vi "Read Response Simple.vi"(7 "output file":path, 8 "error in (no error)":errorcluster, 11 "HttpResponseMessage in":refnum<class "HttpResponseMessage.lvclass">) -> (0 "error out":errorcluster, 1 "Response":string, 2 "Headers":T1, 4 "Timeout":bool, 5 "StatusCode":i32(ring)=100 items=["Continue"=100, "SwitchingProtocols"=101, "OK"=200, "Created"=201, "Accepted"=202, "NonAuthoritativeInformation"=203, "NoContent"=204, "ResetContent"=205, "PartialContent"=206, "MultipleChoices, Ambiguous"=300, "MovedPermanently, Moved"=301, "Found, Redirect"=302, "SeeOther, RedirectMethod"=303, "NotModified"=304, "UseProxy"=305, "Unused"=306, "TemporaryRedirect, RedirectKeepVerb"=307, "BadRequest"=400, "Unauthorized"=401, "PaymentRequired"=402, "Forbidden"=403, "NotFound"=404, "MethodNotAllowed"=405, "NotAcceptable"=406, "ProxyAuthenticationRequired"=407, "RequestTimeout"=408, "Conflict"=409, "Gone"=410, "LengthRequired"=411, "PreconditionFailed"=412, "RequestEntityTooLarge"=413, "RequestUriTooLong"=414, "UnsupportedMediaType"=415, "RequestedRangeNotSatisfiable"=416, "ExpectationFailed"=417, "UpgradeRequired"=426, "InternalServerError"=500, "NotImplemented"=501, "BadGateway"=502, "ServiceUnavailable"=503, "GatewayTimeout"=504, "HttpVersionNotSupported"=505], 6 "ReasonPhrase":string)   [LabVIEW 2018, in "LabVIEWHTTPClient_NET.lvlib" / "HttpResponseMessage.lvclass"]
uses:
  HttpResponseMessage.lvclass
  Types/ResponseHeaders_Cluster.ctl
  HttpHeaders_response/HttpHeaders_Response.lvclass
  HttpHeaders_content/HttpHeaders_Content.lvclass
  HttpContent/HttpContent.lvclass
  LabVIEWHTTPClient_NET/LabVIEWHTTPClient_NET.lvlib
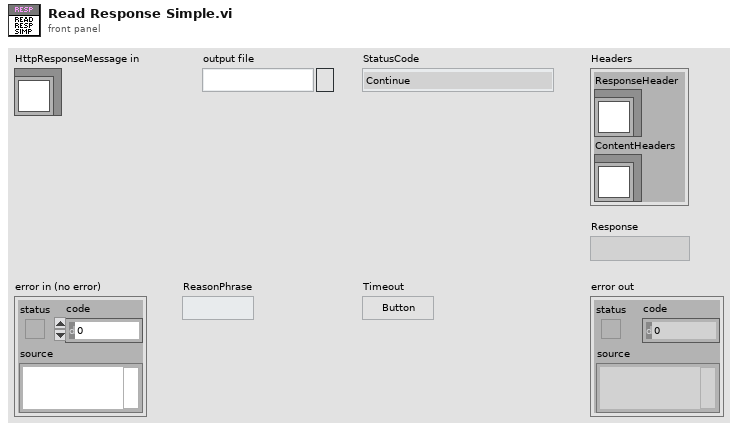
[diagram p1: front panel]
types:
  T1 = typedef "LabVIEWHTTPClient_NET.lvlib/ResponseHeaders_Cluster.ctl" = cluster{"ResponseHeader":refnum<class "HttpHeaders_Response.lvclass">, "ContentHeaders":refnum<class "HttpHeaders_Content.lvclass">}
  T2 = cluster{"HTTPHeaders_NET out":refnum<class "HttpHeaders_Response.lvclass">, "HTTPHeaders":refnum<class "HttpHeaders_Content.lvclass">}
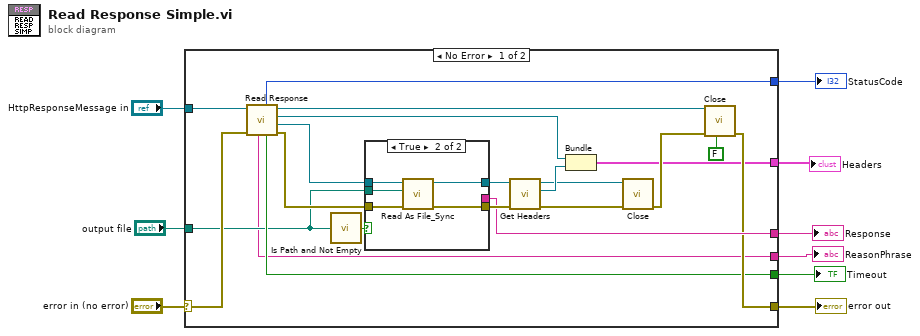
[diagram p0: block diagram]
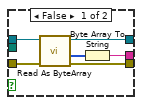
[diagram p2: hidden frame]
diagram:
  n1 = case shown="No Error" "error in (no error)" {
    selector: "error in (no error)" -> [w28 w42]
    tunnel: [w21 w42] -> w8
    tunnel: "HttpResponseMessage in" -> [w27 _]
    tunnel: [w22 _] -> w5
    tunnel: [w20 _] -> w6
    tunnel: [w19 _] -> w3
    tunnel: "output file" -> [w17 _]
    tunnel: [w11 _] -> w2
    tunnel: [w10 _] -> w1
    frame No Error {
      n2 = call "Read Response.vi"("error in (no error)"=w28, "HttpResponseMessage in"=w27) -> ("error out"=w25:errorcluster, "HttpContent out"=w26:refnum<class "HttpContent.lvclass">, "HTTPHeaders_NET out"=w16:refnum<class "HttpHeaders_Response.lvclass">, "HttpResponseMessage out"=w30:refnum<class "HttpResponseMessage.lvclass">, "Timeout"=w20:bool, "StatusCode"=w19:i32, "ReasonPhrase"=w10:string)  [unwired: 3 in]
      n3 = call <vilib>:"Is Path and Not Empty.vi"("path"=w17) -> ("Is Path and Not Empty?"=w18:bool)  [unwired: 4 in]
      n4 = case shown="True" w18 {
        tunnel: w26 -> [w36 w41]
        tunnel: [w34 _] -> w22
        tunnel: w25 -> [w33 w40]
        tunnel: [w32 w39] -> w23
        tunnel: [w31 w38] -> w24
        tunnel: w17 -> [_ w37]
        frame False {
          n5 = call "Read As ByteArray.vi"("error in (no error)"=w33, "HttpContent in"=w36) -> ("error out"=w32:errorcluster, "Content"=w35:u8[], "HttpContent out"=w31:refnum<class "HttpContent.lvclass">)  [unwired: 7 in]
          n6 = Byte Array To String(unsigned byte array=w35) -> (string=w34:string)
        }
        frame True {
          n7 = call "Read As File_Sync.vi"("error in (no error)"=w40, "FilePath"=w37, "HttpContent in"=w41) -> ("error out"=w39:errorcluster, "HttpContent out"=w38:refnum<class "HttpContent.lvclass">)  [unwired: 4 in, 3 out]
        }
      }
      n8 = call "Get Headers.vi"("error in (no error)"=w23, "HttpContent in"=w24) -> ("error out"=w14:errorcluster, "HTTPHeaders"=w15:refnum<class "HttpHeaders_Content.lvclass">, "HttpContent out"=w13:refnum<class "HttpContent.lvclass">)  [unwired: 7 in]
      n9 = Bundle("HTTPHeaders_NET out"=w16, "HTTPHeaders"=w15) -> (w11:T2)  [unwired: 1 in]
      n10 = call "Close.vi"("error in (no error)"=w14, "HttpContent in"=w13) -> ("error out"=w12:errorcluster)  [unwired: 9 in]
      n11 = call "Close.vi"("CloseHeaders"=FALSE, "error in (no error)"=w12, "HttpResponseMessage in"=w30) -> ("error out"=w21:errorcluster)  [unwired: 8 in]
    }
    frame Error {
    }
  }
  "error out" <- w8
  "Timeout" <- w6
  "Response" <- w5
  "StatusCode" <- w3
  "Headers" <- w2
  "ReasonPhrase" <- w1
